vi "Find Object Items by Name.vi"(6 "Item Names":string[](array[string]), 7 "Object Path":string, 8 "error in (no error)":errorcluster, 10 "Starting Offset":i32, 11 "JSON":string) -> (0 "error out":errorcluster, 1 "<JSON>":string[](array[string]) caption="Items<JSON>", 2 "Found":bool[](array[boolean]))   [LabVIEW 2013, in "JSONtext.lvlib"]
doc: "Find multiple Items in a JSON Object, by item names. Output items (as JSON) are in the same order as the supplied item names. If an item is not present, then the output for that item will be an empty string."
uses:
  JSONtext.lvlib
  support/quote and escape json string 2.vi
  Find Item Locations by Path.vi
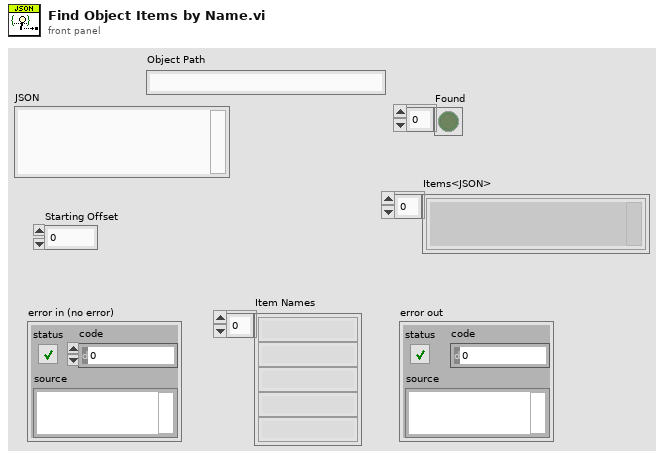
[diagram p1: front panel]
types:
  T1 = typedef "JSONtext.lvlib/Found Items.ctl" = cluster{"Item offset":i32, "Offset past Item":i32, "Name offset":i32, "Offset past Name":i32, "Found":bool, "Empty Object":bool}
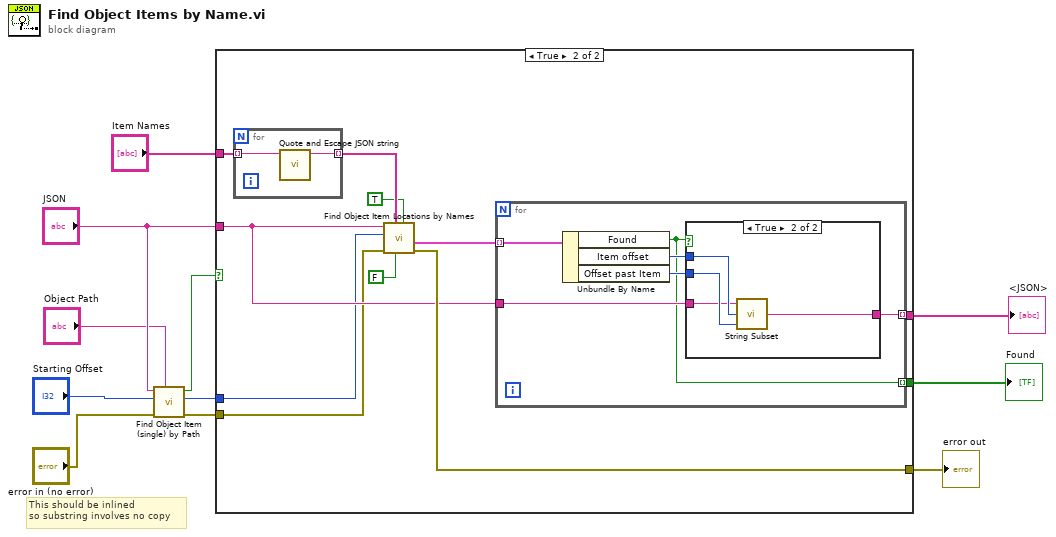
[diagram p0: block diagram]
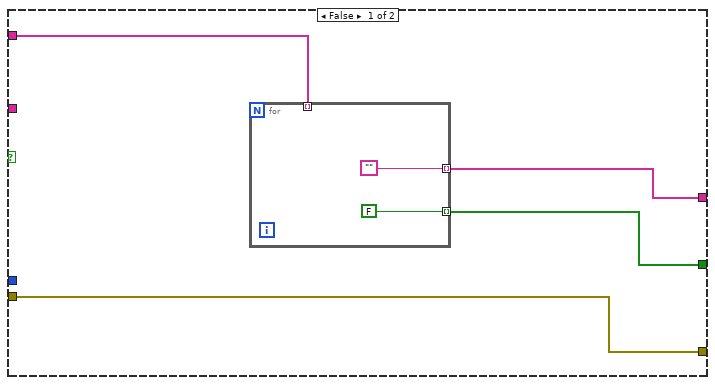
[diagram p2: hidden frame]
diagram:
  # "This should be inlined\nso substring involves no copy"
  n1 = call "Find Object Item (single) by Path.vi"("Item Path"="Object Path", "error in (no error)"="error in (no error)", "Starting Offset"="Starting Offset", "JSON"="JSON") -> ("error out"=w4:errorcluster, "Item offset"=w1:i32, "Found"=w3:bool)  [unwired: 4 in, 1 out]
  n2 = case shown="True" w3 {
    tunnel: [w15 w28] -> w11
    tunnel: [w13 w27] -> w10
    tunnel: "Item Names" -> [w14 w24]
    tunnel: [w12 w21] -> w8
    tunnel: "JSON" -> [_ w20]
    tunnel: w1 -> [_ w19]
    tunnel: w4 -> [w15 w18]
    frame False {
      n3 = for {
        tunnel: w14 -> [_] mode=indexing
        tunnel: [""] -> w13 mode=indexing
        tunnel: [FALSE] -> w12 mode=indexing
      }
    }
    frame True {
      n4 = for {
        tunnel: w24 -> [w30] mode=indexing
        tunnel: [w29] -> w23 mode=indexing
        n5 = call "Quote and Escape JSON string.vi"("Plain Text"=w30) -> ("<JSON>"=w29:string)  [unwired: 10 in]
      }
      n6 = call "Find Object Item Locations by Names.vi"("Insertion point if not found"=TRUE, "Only return first found"=FALSE, "Item Names <JSON>"=w23, "error in (no error)"=w18, "Object Offset"=w19, "JSON"=w20) -> ("error out"=w28:errorcluster, "Items"=w26:T1[])  [unwired: 4 in]
      n7 = for {
        tunnel: w20 -> [w36]
        tunnel: [w35] -> w27 mode=indexing
        tunnel: w26 -> [w32] mode=indexing
        tunnel: [w31] -> w21 mode=indexing
        n8 = Unbundle By Name(w32) -> ("Found"=w31:bool, "Item offset"=w34:i32, "Offset past Item"=w33:i32)
        n9 = case shown="True" w31 {
          tunnel: w36 -> [_ w37]
          tunnel: [_ w40] -> w35
          tunnel: w34 -> [_ w39]
          tunnel: w33 -> [_ w38]
          frame False {
          }
          frame True {
            n10 = call "String Subset.vi"("Offset past End"=w38, "Start offset"=w39, "JSON"=w37) -> ("substring"=w40:string)  [unwired: 2 in]
          }
        }
      }
    }
  }
  "error out" <- w11
  "<JSON>" <- w10
  "Found" <- w8
